vi "Write 7z config.vi"(8 "error in (no error)":errorcluster, 9 "Product Name":string, 10 "Package Version":string, 11 "Package Source Folder":path) -> (0 "error out":errorcluster)   [LabVIEW 2016]
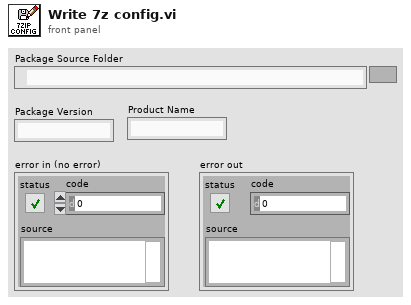
[diagram p1: front panel]
types:
  T1 = enum16{"open", "replace", "create", "open or create", "replace or create", "replace or create with confirmation"}
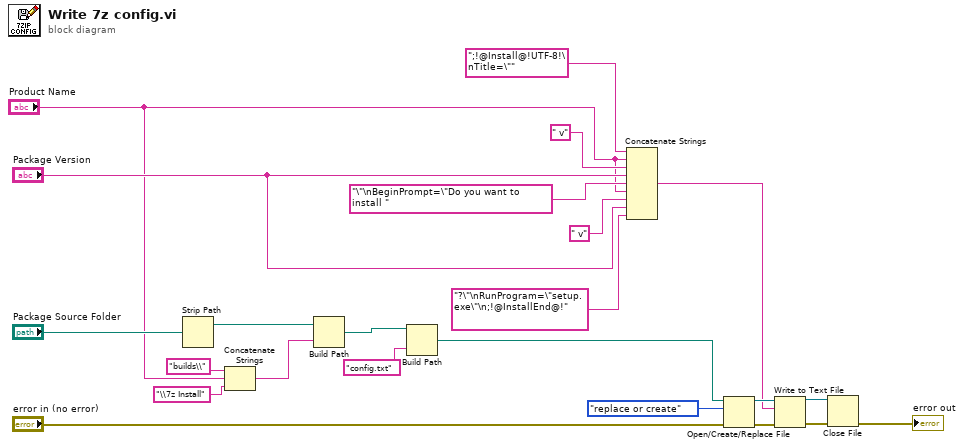
[diagram p0: block diagram]
diagram:
  n1 = Strip Path(path="Package Source Folder") -> (stripped path=w21:path)  [unwired: 1 out]
  n2 = Concatenate Strings("builds\\" ("name or relative path"), "Product Name", "\\7z Install" ("name or relative path")) -> (w1:string)
  n3 = Build Path(base path=w21, name or relative path=w1) -> (appended path=w9:path)
  n4 = Build Path(base path=w9, name or relative path="config.txt") -> (appended path=w14:path)
  n5 = Concatenate Strings(";!@Install@!UTF-8!\nTitle=\"" ("Name of target (My Computer)"), "Product Name", " v" ("Name of target (My Computer)"), "Package Version", "\"\nBeginPrompt=\"Do you want to install " ("Name of target (My Computer)"), "Product Name", " v" ("Name of target (My Computer)"), "Package Version", "?\"\nRunProgram=\"setup.exe\"\n;!@InstallEnd@!" ("Name of target (My Computer)")) -> (w17:string)
  n6 = Open/Create/Replace File(file path (use dialog)=w14, error in="error in (no error)", operation (0:open)=T1."replace or create") -> (refnum out=w18:refnum<file>, error out=w15:errorcluster)  [unwired: 3 in, 1 out]
  n7 = Write to Text File(file (use dialog)=w18, text=w17, error in=w15) -> (refnum out=w11:refnum<file>, error out=w12:errorcluster)  [unwired: 1 in, 1 out]
  n8 = Close File(refnum=w11, error in=w12) -> (error out=→"error out":errorcluster)  [unwired: 1 out]
